vi "Get Short Help.vi"(8 "error in (no error)":errorcluster, 11 "Build in":refnum<class "Build.lvclass">) -> (0 "error out":errorcluster, 2 "Short Help":string, 3 "Build out":refnum<class "Build.lvclass">)   [LabVIEW 2020, in "Build.lvlib" / "Build.lvclass"]
uses:
  Build.lvclass
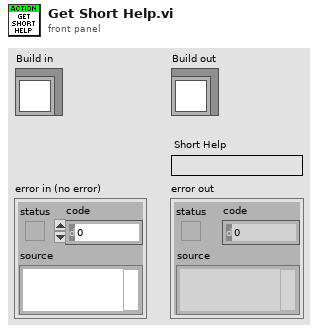
[diagram p1: front panel]
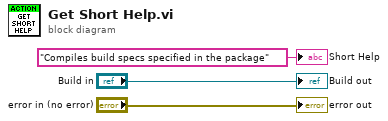
[diagram p0: block diagram]
diagram:
  "error out" <- "error in (no error)"
  "Build out" <- "Build in"
  "Short Help" <- "Compiles build specs specified in the package" ("Short Help")
